vi "Count.vi"(8 "error in (no error)":errorcluster, 11 "List in":refnum<class "ObjectList.lvclass">) -> (0 "error out":errorcluster, 2 "Number of Items":i32, 3 "List out":refnum<class "ObjectList.lvclass">)   [LabVIEW 2013, in "LapDog.Collections.v1.Lists.lvlib" / "ObjectList.lvclass"]
doc: "Returns the number of items currently in the list."
uses:
  ObjectList.lvclass
  ObjectList.lvclass/ObjectList.ctl
  ListImp/ListImp.lvclass
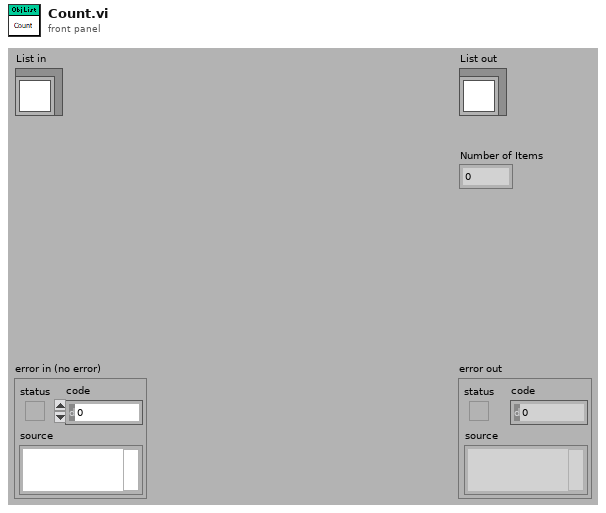
[diagram p1: front panel]
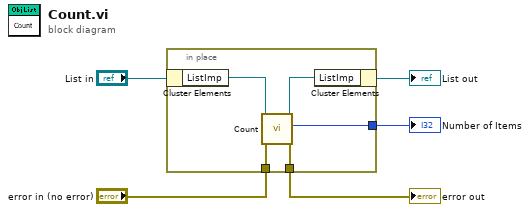
[diagram p0: block diagram]
diagram:
  n1 = in-place {
    in-place-border: [w10] -> w1
    in-place-border: "error in (no error)" -> [w9]
    in-place-border: [w8] -> w4
    n2 = in-place-cluster #1("List in") -> ("ListImp"=w7:refnum<class "ListImp.lvclass">)
    n3 = call-dynamic "Count.vi"("error in (no error)"=w9, "ListImp in"=w7) -> ("error out"=w8:errorcluster, "Number of Items"=w10:i32, "ListImp out"=w6:refnum<class "ListImp.lvclass">)  [unwired: 7 in]
    n4 = in-place-cluster #1("ListImp"=w6) -> (→"List out":refnum<class "ObjectList.lvclass">)
  }
  "error out" <- w4
  "Number of Items" <- w1
